vi "3D Drift Control.vi"() -> ()   [LabVIEW 2010]
uses:
  <vilib>/Analysis/NI_AALBase.lvlib
panel:
  out "Boolean":bool
  out "date string":string
  in  "date format (0)":enum16{"short", "long", "abbreviated"}(ring)
  in  "Reset":bool
  in  "# Average":i32=1 min=1 max=20 step=1
  in  "Position (um)":dbl=5.0 min=0.0 max=12.0 format="%0.2f"
  in  "Center Piezo":bool
  in  "reset":bool
  out "?":bool
  in  "autofocus":bool
  out "afTemplateImg":dbl[][](array[numeric])
  in  "Select Lockin \n(autofocus)":bool
  out "Image":u8[][](graph)
  out "ztemplateImg":dbl[][](array[numeric])
  in  "z-template":dbl=0.8
  out "z-sensitivity":dbl
  in  "P (z)":dbl=0.1
  in  "I (z)":dbl=0.0005
  out "z-setpoint":dbl
  in  "z-window (um)":dbl=0.5
  in  "z-stepsiz (um)":dbl=0.1
  out "Step":i32
  in  "Save Data":bool
  out "Total Steps":dbl
  in  "stop":bool
  in  "Exposure time 2":dbl(slide)=16.823708333333332 min=0.06254166666666666 max=66.66941666666666 step=0.06254166666666666 scale=0.06254166666666666..103.94425 scale format="%#.3g"
  in  "Pixel clock":i32(slide)=24 min=5 max=40 scale=5.0..40.0
  in  "Frame rate":dbl(slide)=50.0 min=0.47316940221670395 max=14.999381275522385 step=6.254166666666666e-05 scale=0.47316940221670395..50.0 scale format="%^#_3g"
  in  "?":bool
  in  "pixels2um":dbl=9.8472
  in  "fix z":bool
  in  "fix y":bool
  in  "fix x":bool
  in  "I (xy)":dbl=0.0005
  in  "P (xy)":dbl=0.1
  out "# of frames":i32
  out "?":cluster{"Y":dbl[], "Y":dbl[]}[](graph)
  in  "Monitor Drift":bool
  out "status":dbl
  out "lockinImg":dbl[][](array[numeric])
  out "centery":dbl
  out "centerx":dbl
  out "?":bool
  in  "Select Lockin\n(Drift Bead)":bool
  in  "templateSiz":dbl=50.0
  in  "add Factor":dbl=20.0
  in  "scale":dbl=9.0
  in  "Filename":string="Drift"
  in  "Index #":i32=1
  out "X Position":dbl
  out "Y Position":dbl
  out "Z Position":dbl
  # "drift"
  # "autofocus"
  # "O"
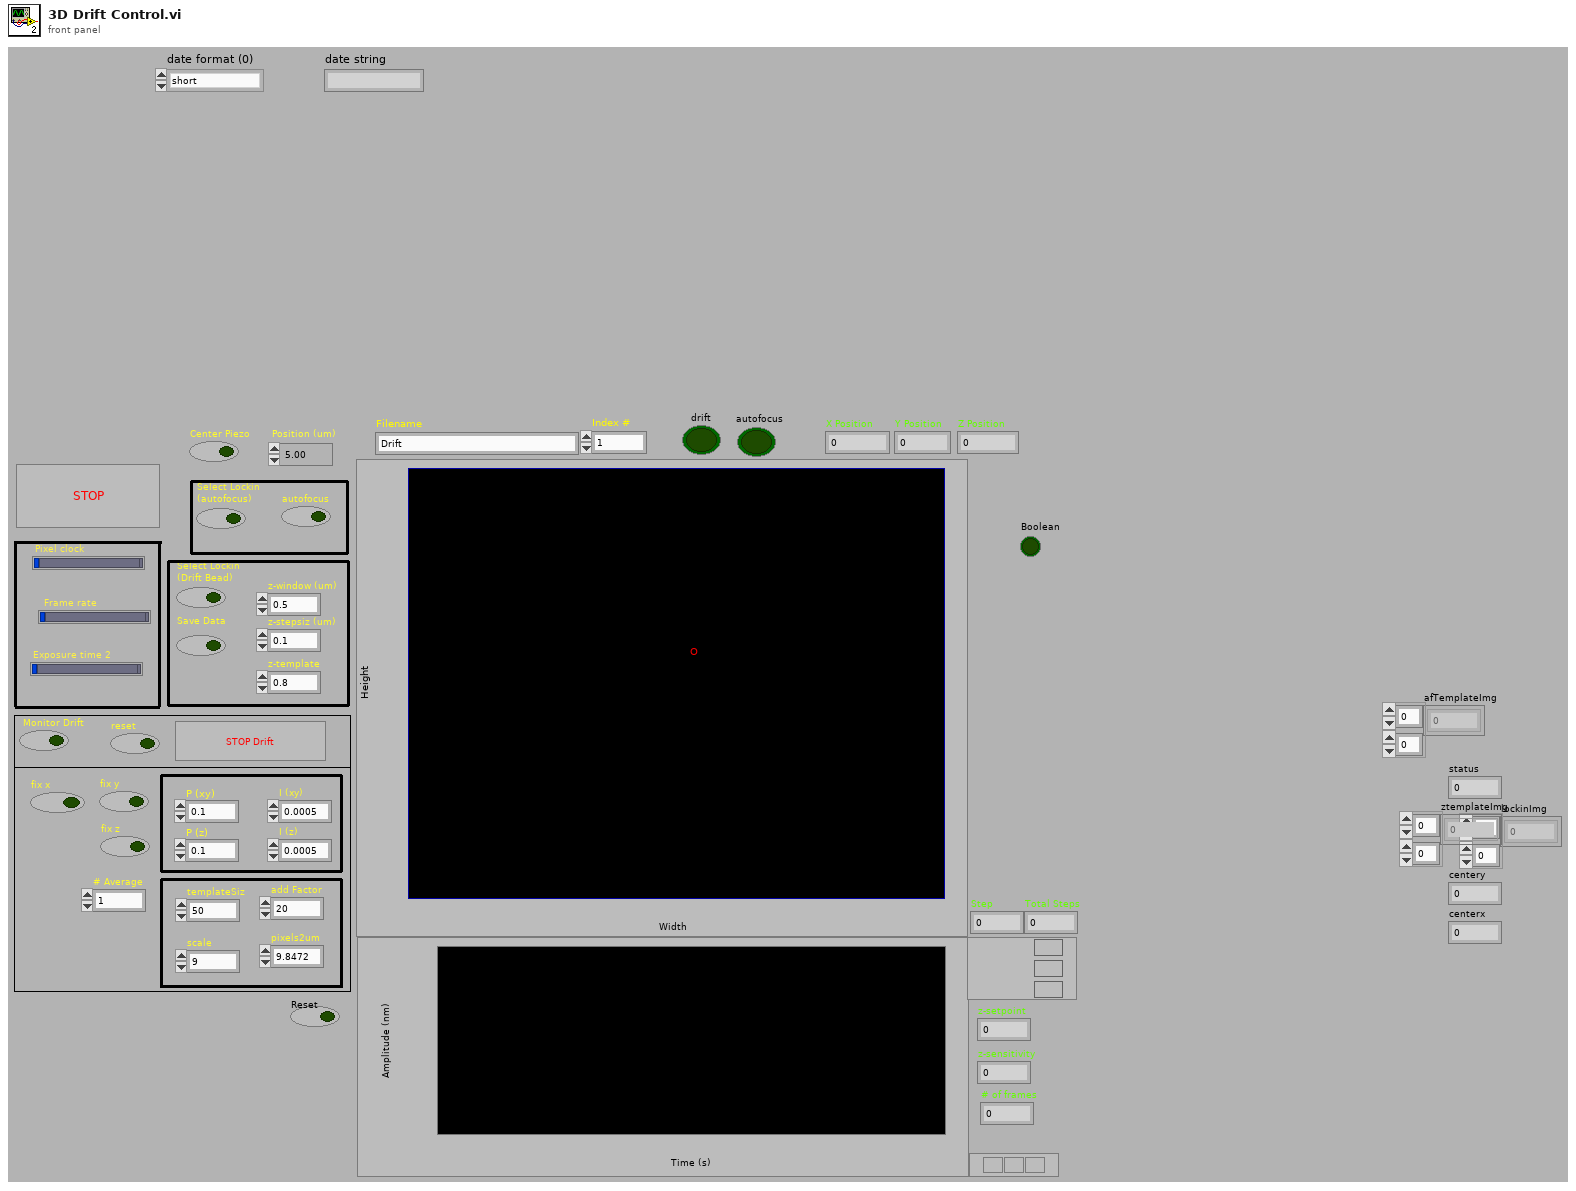
[diagram p1: front panel]
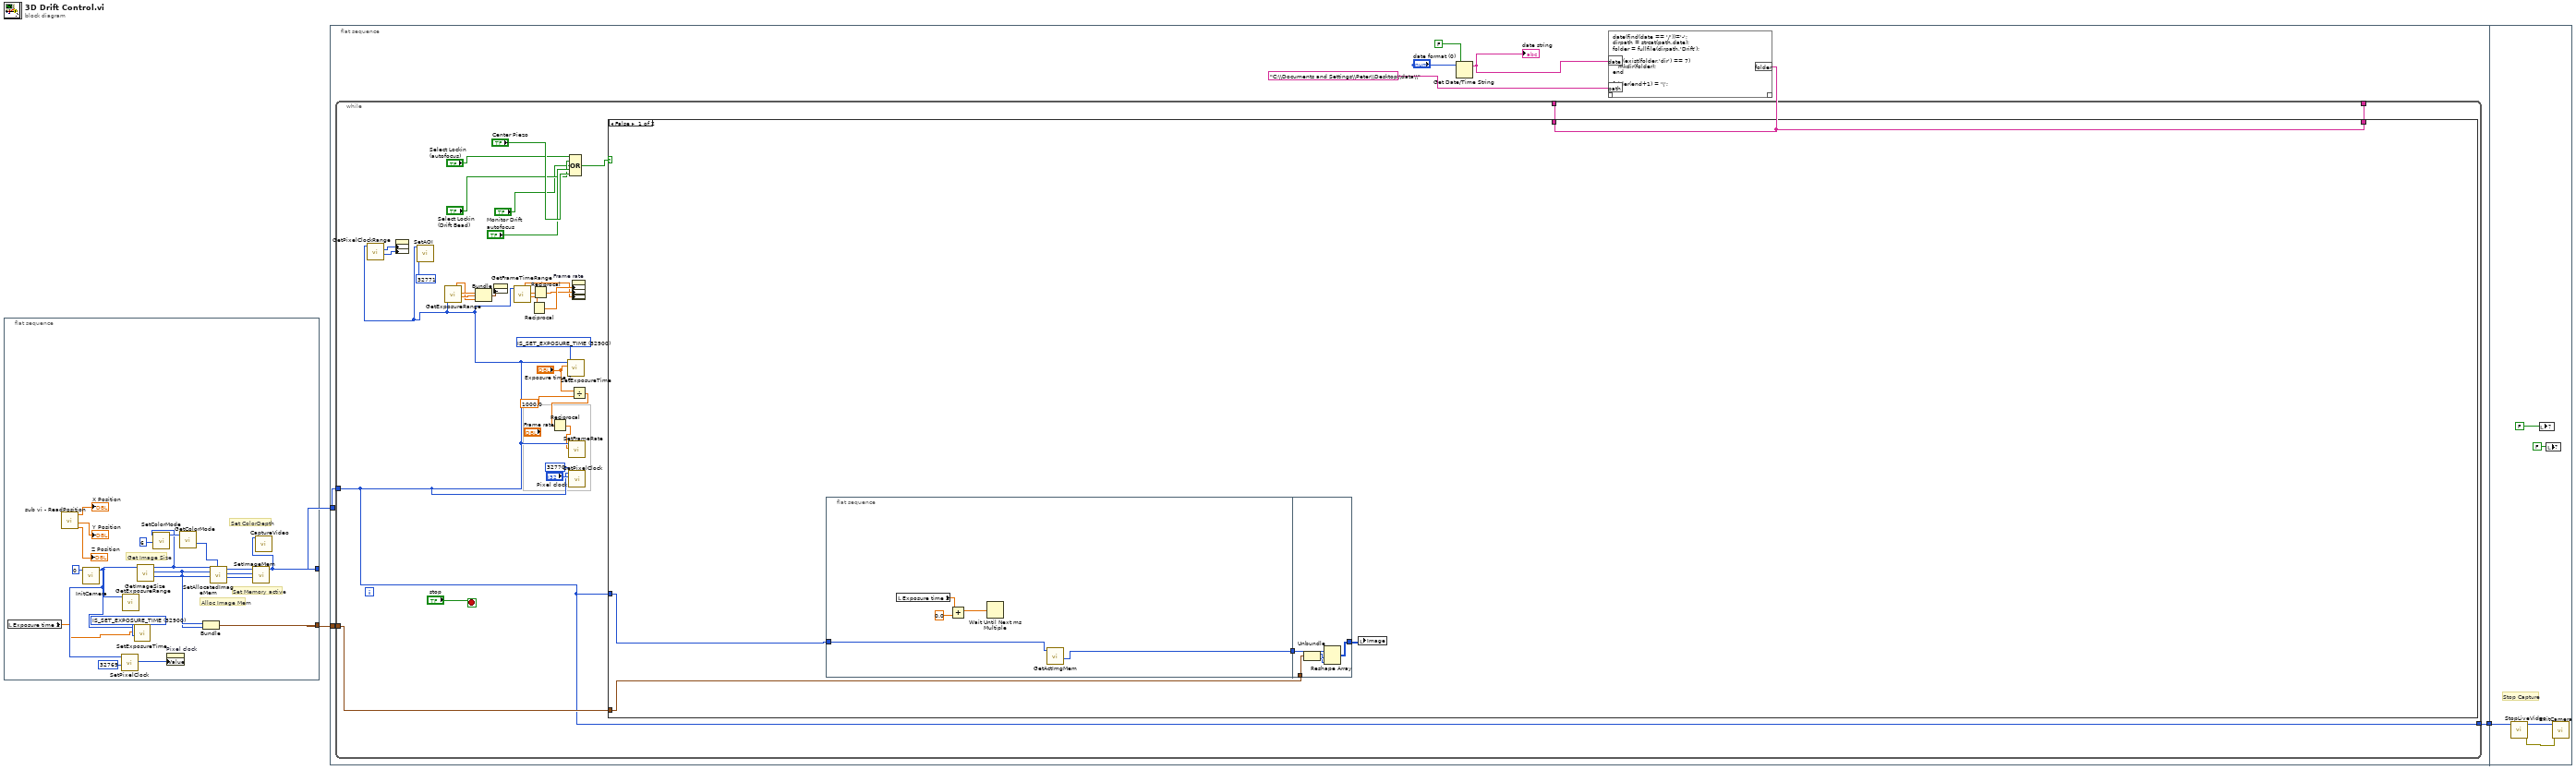
[diagram p0: block diagram]
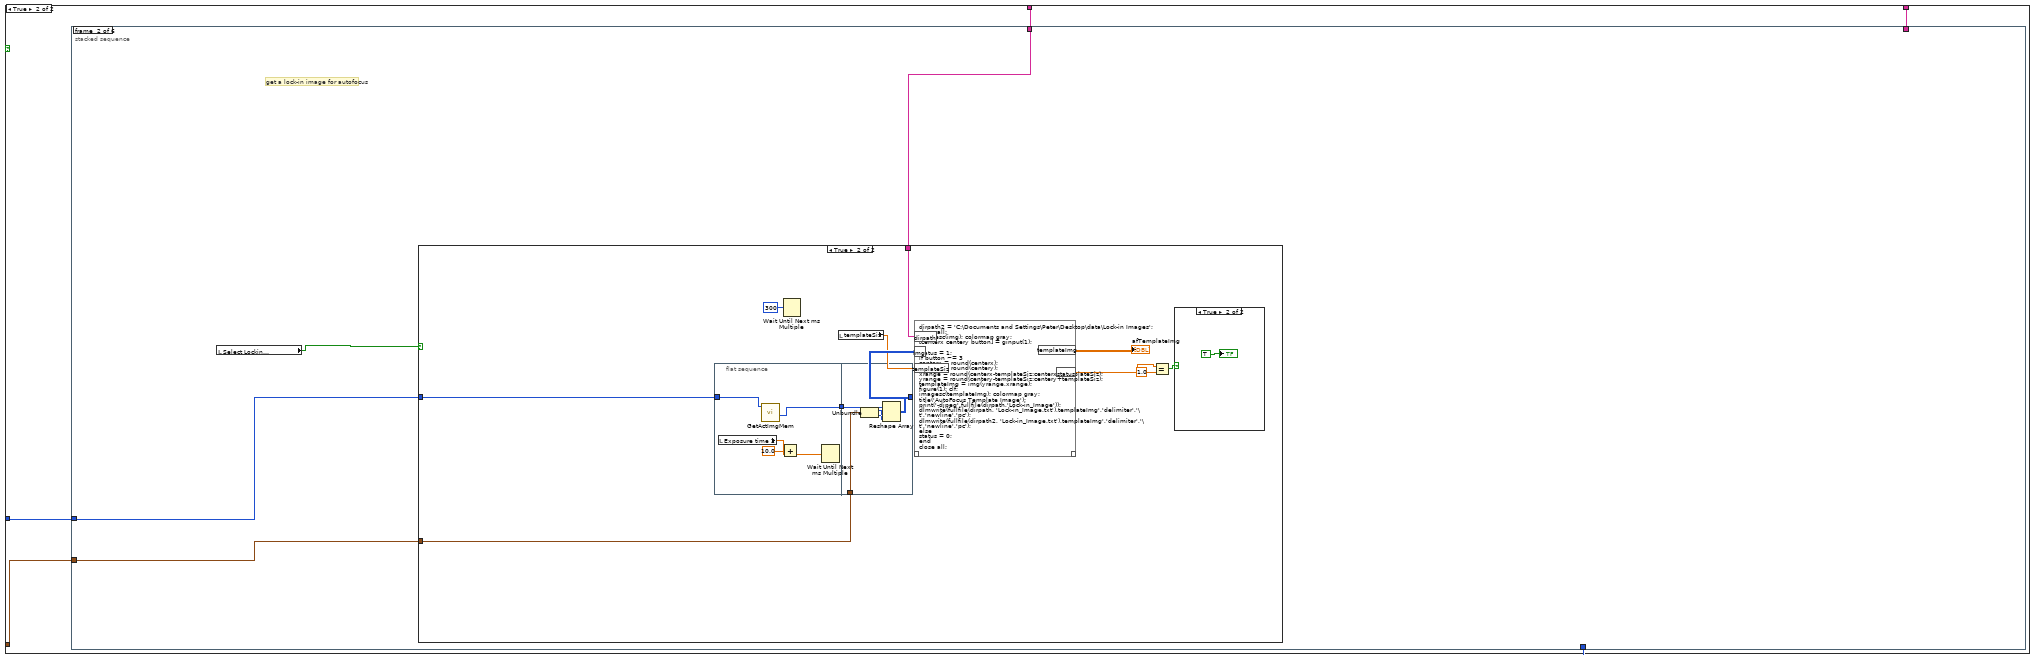
[diagram p2: hidden frame]
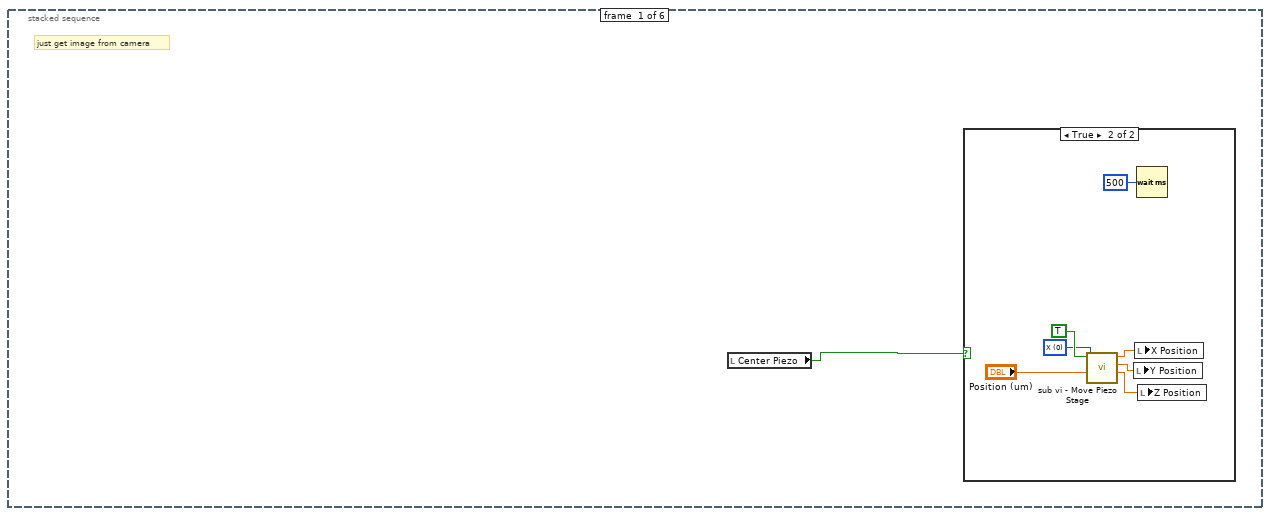
[diagram p3: hidden frame]
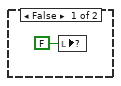
[diagram p6: hidden frame]
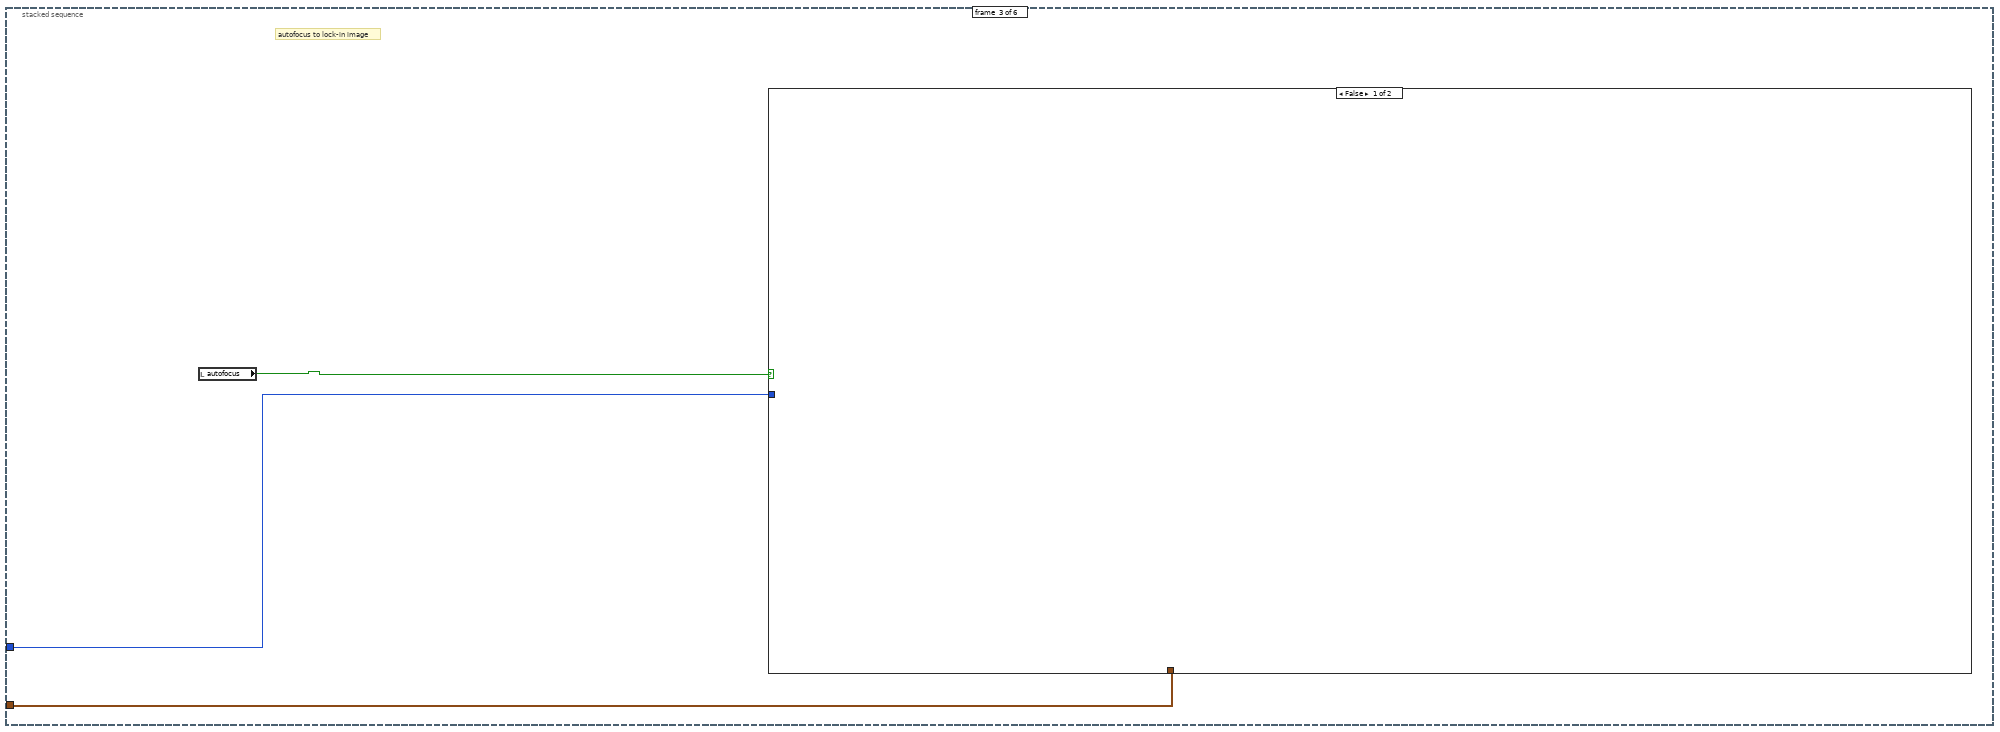
[diagram p7: hidden frame]
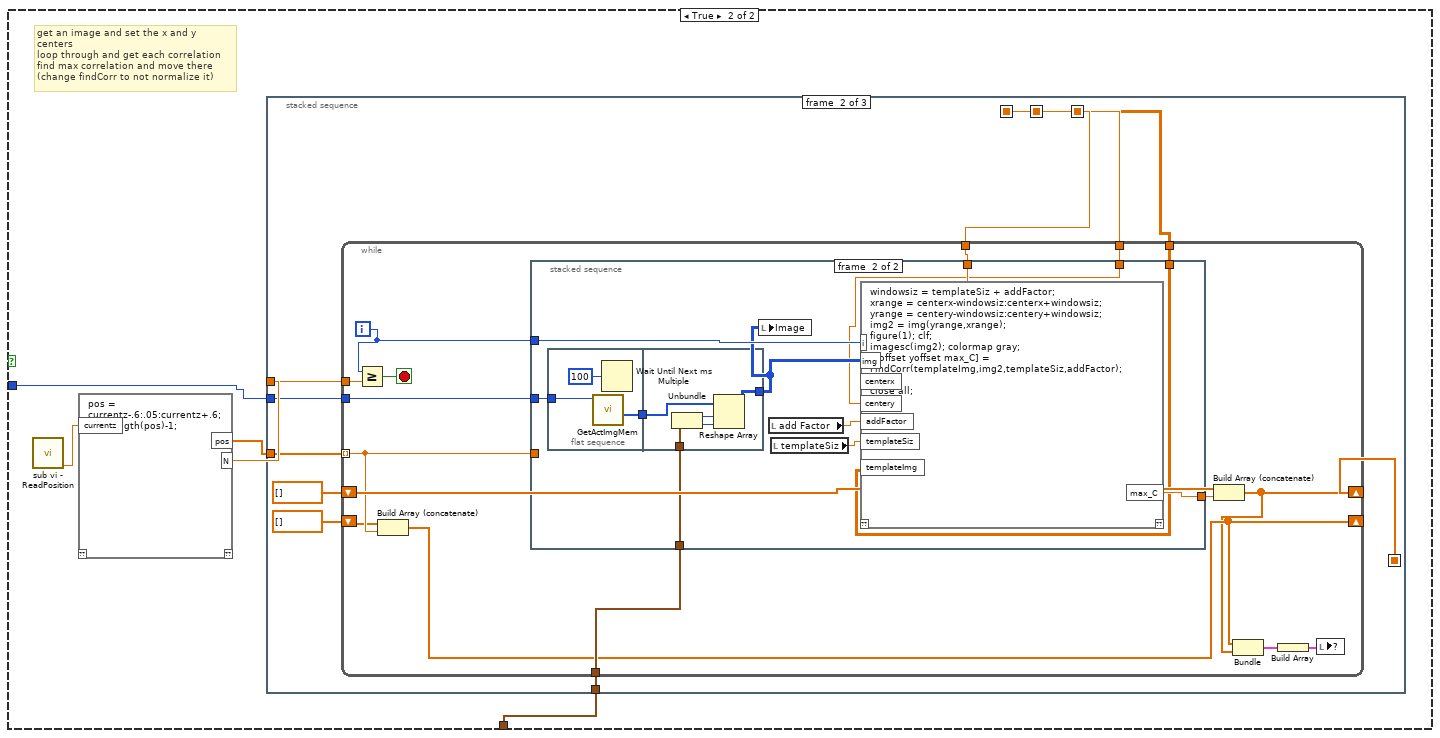
[diagram p8: hidden frame]
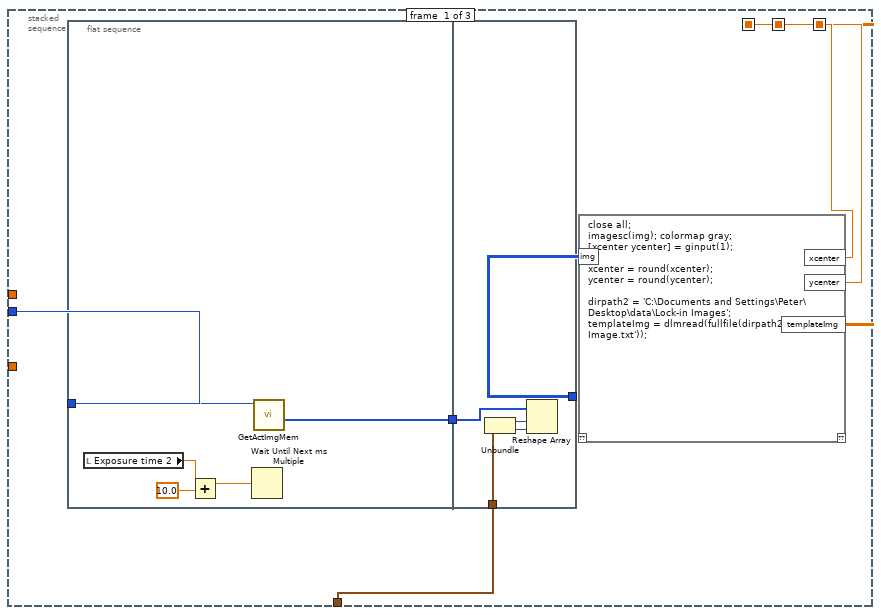
[diagram p9: hidden frame]
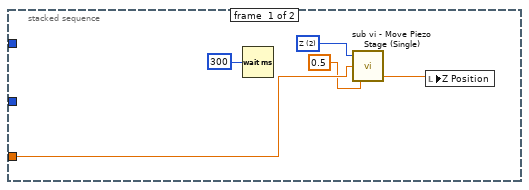
[diagram p10: hidden frame]
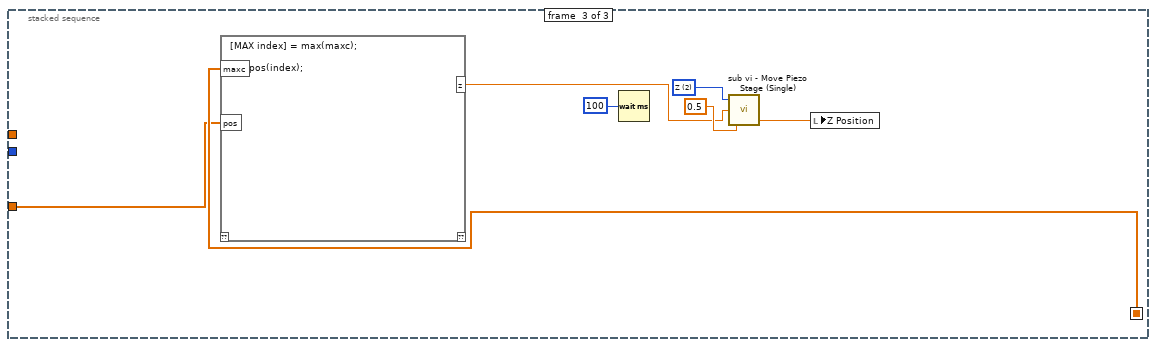
[diagram p11: hidden frame]
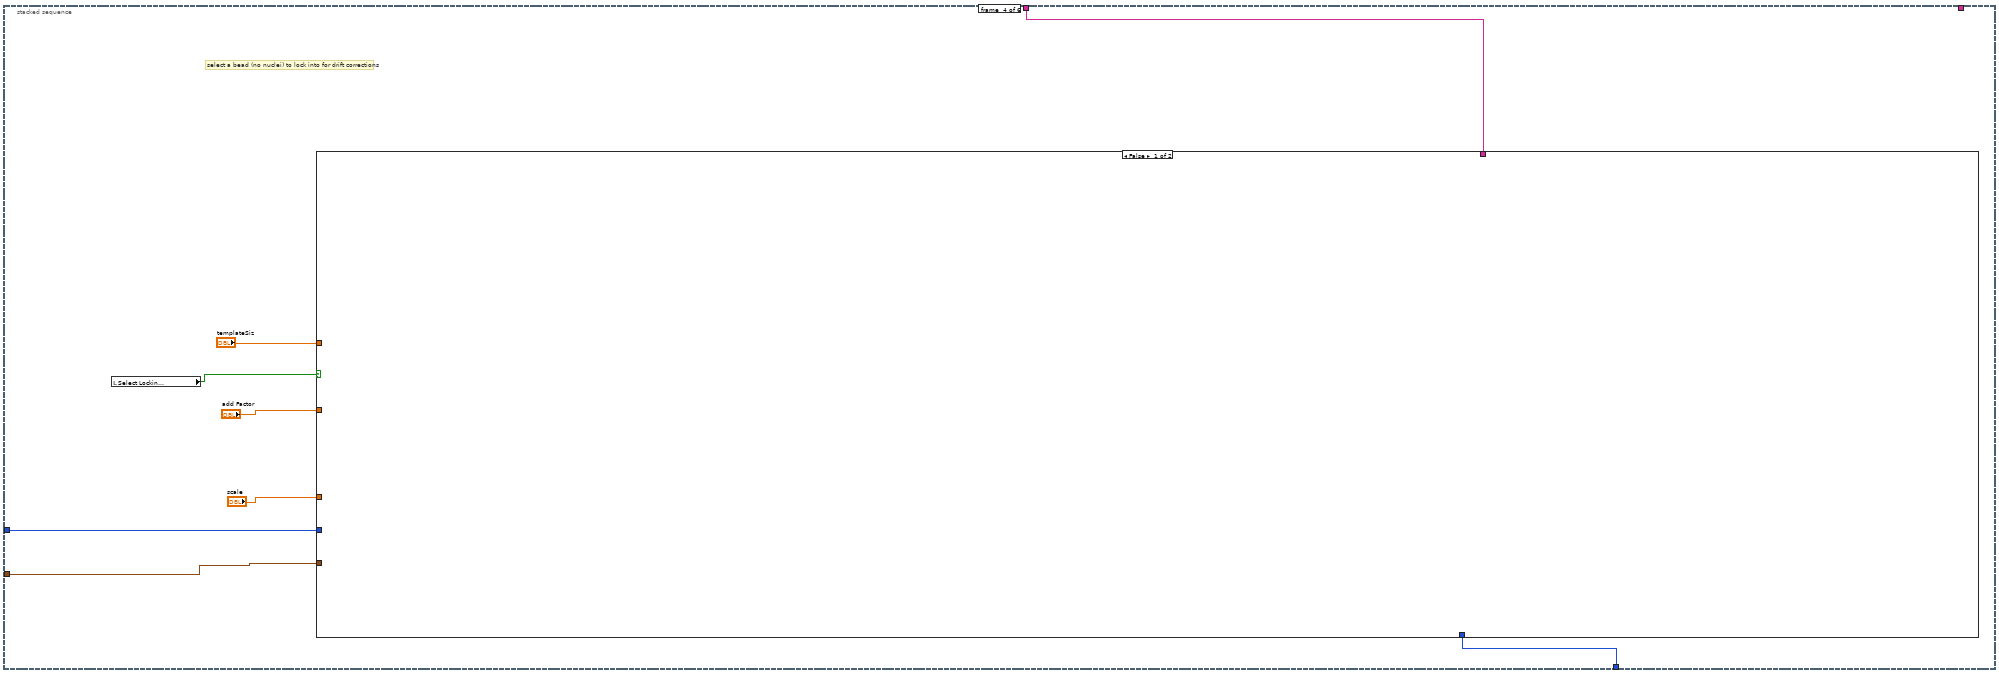
[diagram p12: hidden frame]
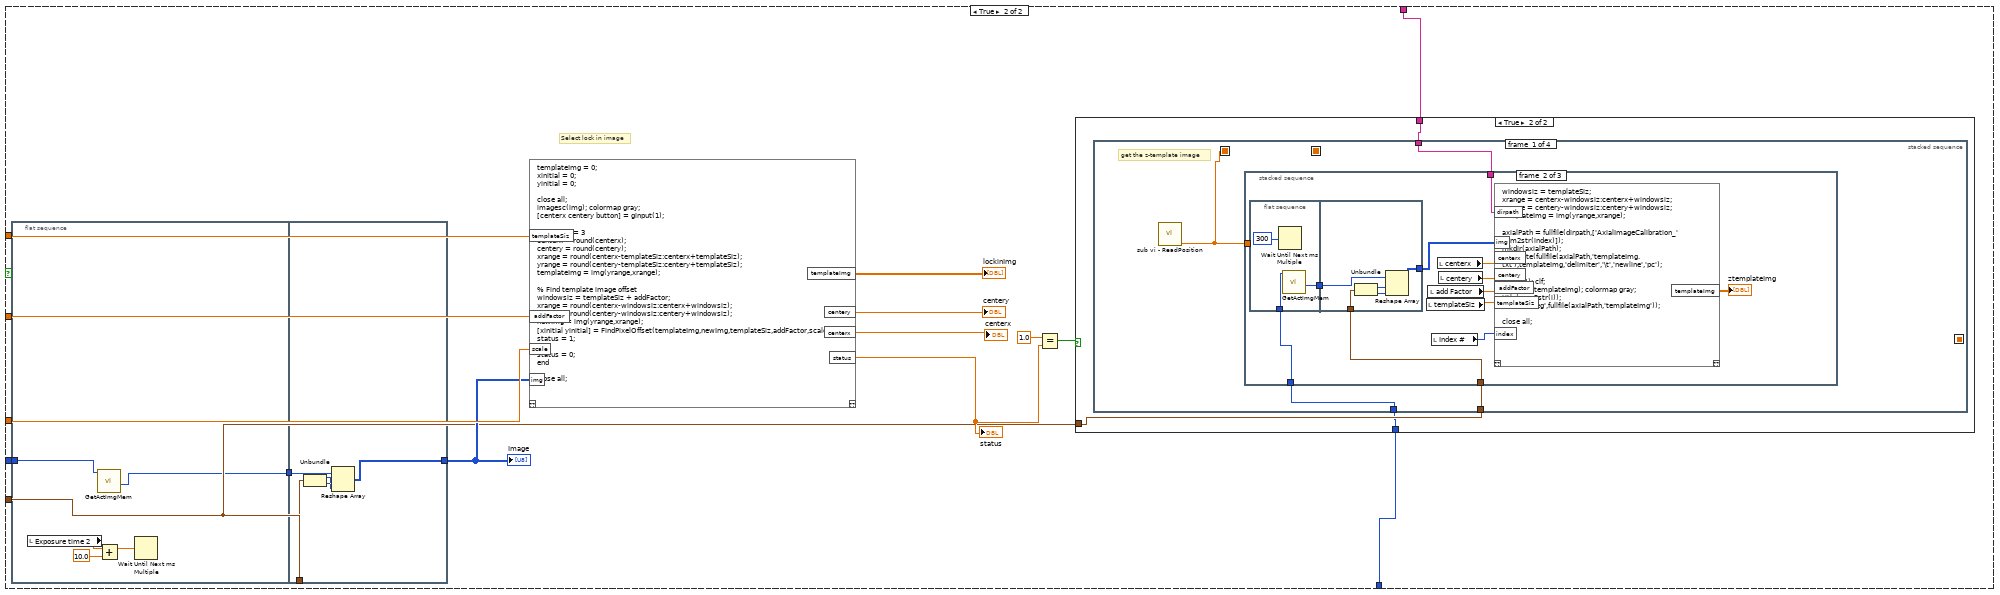
[diagram p13: hidden frame]
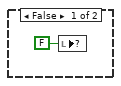
[diagram p14: hidden frame]
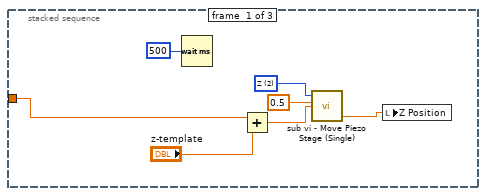
[diagram p15: hidden frame]
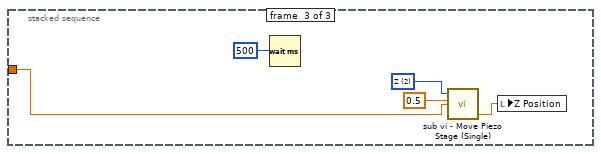
[diagram p16: hidden frame]
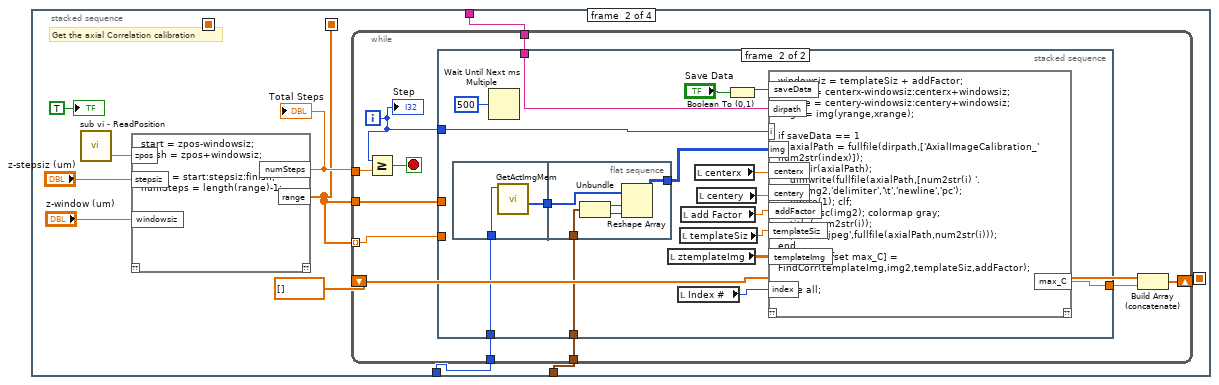
[diagram p17: hidden frame]
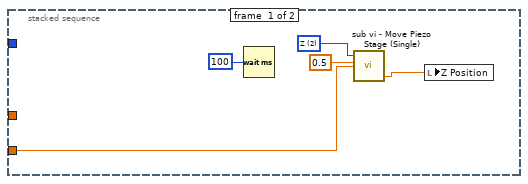
[diagram p18: hidden frame]
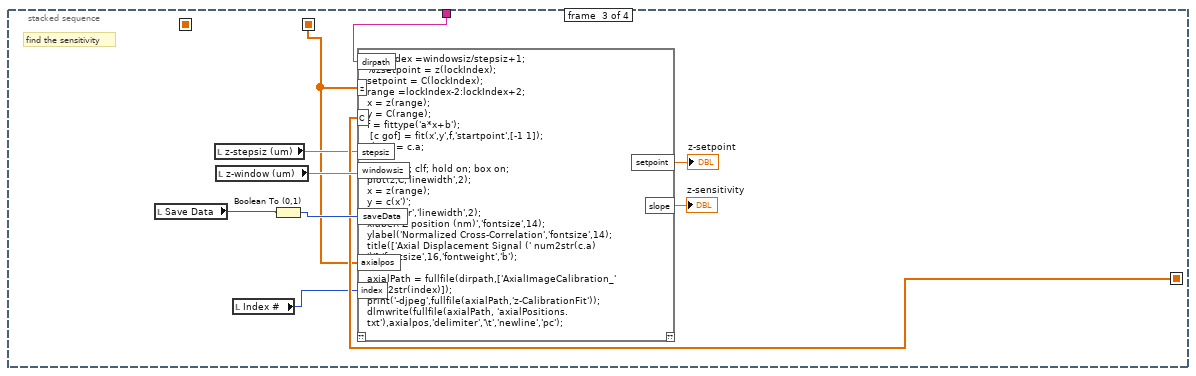
[diagram p19: hidden frame]
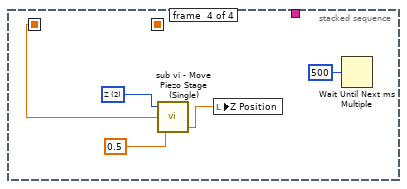
[diagram p20: hidden frame]
diagram:
  n1 = flat-sequence {
    tunnel: [w6] -> w2
    tunnel: [w9] -> w1
    frame #0 {
      w11 = u16 32900 items=["IS_SET_EXPOSURE_TIME"=32900, "IS_GET_EXPOSURE_TIME"=32768, "IS_GET_DEFAULT_EXPOSURE"=32769] ("Mode")
      # "Set Memory active"
      # "Alloc Image Mem"
      # "Set ColorDepth"
      # "Get Image Size"
      n2 = local read "Exposure time 2"() -> (w7:dbl)
      n3 = call "sub vi - ReadPosition.vi"() -> ("Z Position"=→"Z Position":dbl, "Y Position"=→"Y Position":dbl, "X Position"=→"X Position":dbl)  [unwired: 6 in, 3 out]
      n4 = call "InitCamera.vi"("Camera ID"=u32 0) -> ("Camera Handle Out"=w10:u32)  [unwired: 10 out]
      n5 = call "SetPixelClock.vi"("Mode"=32769, "Camera Handle In"=w10) -> ("Value"=w8:i32)  [unwired: 2 in, 7 out]
      n6 = call "GetExposureRange.vi"("Camera Handle In"=w10) -> ()  [unwired: 1 in, 10 out]
      n7 = call "SetExposureTime.vi"("Mode"=w11, "Exposure Time"=w7, "Camera Handle In"=w10) -> ()  [unwired: 2 in, 7 out]
      n8 = call "GetImageSize.vi"("Camera Handle In"=w10) -> ("Height"=w13:i32, "Width"=w12:i32, "Camera Handle Out"=w4:u32)  [unwired: 8 out]
      n9 = call "SetColorMode.vi"("Mode"=6, "Camera Handle In"=w4) -> ("Camera Handle Out"=w16:u32)  [unwired: 1 in, 8 out]
      n10 = property on="Pixel clock" class="Slide (strict)"("Value"=w8) -> ()  [unwired: 2 in, 2 out]
      n11 = call "GetColorMode.vi"("Camera Handle In"=w16) -> ("Bits/Pixel"=w14:i32)  [unwired: 10 out]
      n12 = Bundle("Height"=w13, "Width"=w12) -> (w9:cluster{"Height":i32, "Width":i32})  [unwired: 1 out]
      n13 = call "SetAllocatedImageMem.vi"("BitsPixel"=w14, "Height"=w13, "Width"=w12, "Camera Handle In"=w4) -> ("Image Memory Out"=w18:u8[], "Memory ID Out"=w19:i32, "Camera Handle Out"=w20:u32)  [unwired: 1 in, 4 out]
      n14 = call "SetImageMem.vi"("Image Memory In"=w18, "Memory ID In"=w19, "Camera Handle In"=w20) -> ("Camera Handle Out"=w6:u32)  [unwired: 1 in, 7 out]
      n15 = call "CaptureVideo.vi"("Camera Handle In"=w6) -> ()  [unwired: 2 in, 9 out]
    }
  }
  n16 = flat-sequence {
    tunnel: w2 -> [w31]
    tunnel: w1 -> [w30]
    tunnel: [w29] -> w3
    tunnel: w3 -> [w558]
    frame #0 {
      n17 = Get Date/Time String(date format (0)="date format (0)", want seconds? (F)=FALSE) -> (date string=w26:string)  [unwired: 2 out]
      "date string" <- w26
      n18 = script code="date(find(date == '/'))='-';\ndirpath = strcat(path,date);\nfolder = fullfile(dirpath,'Drift');\n\nif ~(exist(folder,'dir') == 7)\n   mkdir(folder);\nend\n\nfolder(end+1) = '\\';"("date"=w26, "path"="C:\\Documents and Settings\\Peter\\Desktop\\data\\" ("String")) -> ("folder"=w24:string)  [unwired: 2 out]
      n19 = while {
        tunnel: w31 -> [w42]
        tunnel: w30 -> [w57]
        tunnel: [w42] -> w29
        tunnel: w24 -> [w56]
        tunnel: w24 -> [w55]
        stop <- "stop" stop-if-true
        w59 = u16 32900 items=["IS_SET_EXPOSURE_TIME"=32900, "IS_GET_EXPOSURE_TIME"=32768, "IS_GET_DEFAULT_EXPOSURE"=32769] ("Mode")
        n20 = call "GetPixelClockRange.vi"("Camera Handle In"=w42) -> ("Max"=w54:i32, "Min"=w53:i32)  [unwired: 1 in, 8 out]
        n21 = property on="Pixel clock" class="Schieberegler (strikt)"("Minimum"=w53, "Maximum"=w54) -> ()  [unwired: 2 in, 2 out]
        n22 = call "SetAOI.vi"("Camera Handle In"=w42, "Mode"=32771) -> ()  [unwired: 5 in, 9 out]
        n23 = call "GetExposureRange.vi"("Camera Handle In"=w42) -> ("max"=w49:dbl, "min"=w50:dbl, "intervall"=w48:dbl)  [unwired: 1 in, 7 out]
        n24 = Bundle("min"=w50, "max"=w49, "intervall"=w48) -> (w51:cluster{"min":dbl, "max":dbl, "intervall":dbl})  [unwired: 1 out]
        n25 = property on="Exposure time 2" class="Schieberegler (strikt)"("Data Range"=w51) -> ()  [unwired: 2 in, 2 out]
        n26 = call "GetFrameTimeRange.vi"("Camera Handle In"=w42) -> ("max"=w47:dbl, "min"=w46:dbl, "interval"=w43:dbl)  [unwired: 1 in, 7 out]
        n27 = Reciprocal(x=w47) -> (1/x=w45:dbl)
        n28 = Reciprocal(x=w46) -> (1/x=w44:dbl)
        n29 = call "SetExposureTime.vi"("Mode"=w59, "Exposure Time"="Exposure time 2", "Camera Handle In"=w42) -> ()  [unwired: 1 in, 8 out]
        n30 = call "SetPixelClock.vi"("Mode"=32770, "Pixel Clock"="Pixel clock", "Camera Handle In"=w42) -> ()  [unwired: 1 in, 8 out]
        n31 = Compound Arithmetic op=OR("Select Lockin \n(autofocus)", "Select Lockin\n(Drift Bead)", "Monitor Drift", "autofocus", "Center Piezo") -> (w37:bool)
        n32 = Divide(x="Exposure time 2", y=1000.0) -> (x/y=w38:dbl)
        n33 = Reciprocal(x=w38) -> (1/x=w41:dbl)
        n34 = call "SetFrameRate.vi"("FPS"=w41, "Camera Handle In"=w42) -> ()  [unwired: 1 in, 9 out]
        n35 = property on="Frame rate" class="Schieberegler (strikt)"("Minimum"=w45, "Maximum"=w44, "Increment"=w43) -> ()  [unwired: 2 in, 2 out]
        n36 = case shown="False" w37 {
          tunnel: w57 -> [w62 w79]
          tunnel: w56 -> [_ w78]
          tunnel: w55 -> [_ w77]
          tunnel: w42 -> [w63 w76]
          frame False {
            n37 = flat-sequence {
              tunnel: [w70] -> w65
              tunnel: w63 -> [w66]
              tunnel: w65 -> [w75]
              tunnel: w62 -> [w74]
              tunnel: [w71] -> w64
              frame #0 {
                n38 = local read "Exposure time 2"() -> (w69:dbl)
                n39 = Add(x=w69, y=0.0) -> (x+y=w68:dbl)
                n40 = Wait Until Next ms Multiple(millisecond multiple=w68) -> ()  [unwired: 1 out]
                n41 = call "GetActImgMem.vi"("Camera Handle In"=w66) -> ("Image Memory Out"=w70:u8[])  [unwired: 1 in, 9 out]
              }
              frame #1 {
                n42 = Unbundle(w74) -> ("Height"=w73:i32, "Width"=w72:i32)
                n43 = Reshape Array(w75, w73, w72) -> (w71:u8[][])
              }
            }
            n44 = local write "Image"(w64) -> ()
          }
          frame True {
            n45 = stacked-sequence {
              tunnel: w76 -> [_ w91 w116 w198 w339 _]
              tunnel: w79 -> [_ w90 w117 w199 w340 _]
              tunnel: w78 -> [_ w89 _ w201 _ _]
              tunnel: w76 -> [_ _ _ w200 _ _]
              tunnel: w77 -> [_ _ _ _ w335 _]
              frame #0 {
                # "just get image from camera"
                n46 = local read "Center Piezo"() -> (w80:bool)
                n47 = case shown="True" w80 {
                  frame False {
                  }
                  frame True {
                    w86 = u16 0 items=["X", "Y", "Z"] ("Axis")
                    n48 = call "sub vi - Move Piezo Stage.vi"("Desired Position (um)"="Position (um)", "Axis"=w86, "All Axis"=TRUE) -> ("Z Position"=w83:dbl, "Y Position"=w84:dbl, "X Position"=w85:dbl)  [unwired: 6 in]
                    n49 = local write "Y Position"(w84) -> ()
                    n50 = local write "X Position"(w85) -> ()
                    n51 = Wait (ms)(milliseconds to wait=u32 500) -> ()  [unwired: 1 out]
                    n52 = local write "Z Position"(w83) -> ()
                  }
                }
              }
              frame #1 {
                # "get a lock-in image for autofocus"
                n53 = local read "Select Lockin \n(autofocus)"() -> (w88:bool)
                n54 = case shown="True" w88 {
                  tunnel: w91 -> [_ w101]
                  tunnel: w90 -> [_ w100]
                  tunnel: w89 -> [_ w99]
                  frame False {
                  }
                  frame True {
                    n55 = flat-sequence {
                      tunnel: [w109] -> w102
                      tunnel: w101 -> [w108]
                      tunnel: w102 -> [w114]
                      tunnel: w100 -> [w113]
                      tunnel: [w110] -> w98
                      frame #0 {
                        n56 = local read "Exposure time 2"() -> (w107:dbl)
                        n57 = call "GetActImgMem.vi"("Camera Handle In"=w108) -> ("Image Memory Out"=w109:u8[])  [unwired: 1 in, 9 out]
                        n58 = Add(x=10.0, y=w107) -> (x+y=w106:dbl)
                        n59 = Wait Until Next ms Multiple(millisecond multiple=w106) -> ()  [unwired: 1 out]
                      }
                      frame #1 {
                        n60 = Unbundle(w113) -> ("Height"=w112:i32, "Width"=w111:i32)
                        n61 = Reshape Array(w114, w112, w111) -> (w110:u8[][])
                      }
                    }
                    n62 = Wait Until Next ms Multiple(millisecond multiple=u32 300) -> ()  [unwired: 1 out]
                    n63 = local read "templateSiz"() -> (w96:dbl)
                    n64 = script code="dirpath2 = 'C:\\Documents and Settings\\Peter\\Desktop\\data\\Lock-in Images';\nclose all;\nimagesc(img); colormap gray;\n[centerx centery button] = ginput(1);\n\nstatus = 1;\nif button ~= 3\ncenterx = round(centerx);\ncentery = round(centery);\nxrange = round(centerx-templateSiz:centerx+templateSiz);\nyrange = round(centery-templateSiz:centery+templateSiz);\ntemplateImg = img(yrange,xrange);\nfigure(1); clf;\nimagesc(templateImg); colormap gray;\ntitle('AutoFocus Template Image');\nprint('-djpeg',fullfile(dirpath,'Lock-in_Image'));\ndlmwrite(fullfile(dirpath, 'Lock-in_Image.txt'),templateImg','delimiter','\\t','newline','pc');\ndlmwrite(fullfile(dirpath2, 'Lock-in_Image.txt'),templateImg','delimiter','\\t','newline','pc');\nelse\nstatus = 0;\nend\nclose all;"("dirpath"=w99, "img"=w98, "templateSiz"=w96) -> ("templateImg"=→"afTemplateImg":dbl[][], "status"=w94:dbl)  [unwired: 1 in, 1 out]
                    n65 = Equal?(x=w94, y=1.0) -> (x = y?=w93:bool)
                    n66 = case shown="True" w93 {
                      frame False {
                        n67 = local write item#43(FALSE) -> ()
                      }
                      frame True {
                        "?" <- TRUE
                      }
                    }
                  }
                }
              }
              frame #2 {
                # "autofocus to lock-in image"
                n68 = local read "autofocus"() -> (w115:bool)
                n69 = case shown="False" w115 {
                  tunnel: w117 -> [_ w122]
                  tunnel: w116 -> [_ w121]
                  frame False {
                  }
                  frame True {
                    # "get an image and set the x and y centers\nloop through and get each correlation\nfind max correlation and move there\n(change findCorr to not normalize it)"
                    n70 = call "sub vi - ReadPosition.vi"() -> ("Z Position"=w120:dbl)  [unwired: 6 in, 5 out]
                    n71 = script code="pos = currentz-.6:.05:currentz+.6;\nN = length(pos)-1;"("currentz"=w120) -> ("pos"=w119:dbl[], "N"=w118:dbl)  [unwired: 1 in, 1 out]
                    n72 = stacked-sequence {
                      seq-local: [w125 _ _] -> [_ w145 _]
                      seq-local: [w124 _ _] -> [_ w144 _]
                      seq-local: [_ w143 _] -> [_ _ w196]
                      seq-local: [w123 _ _] -> [_ w140 _]
                      tunnel: w122 -> [w128 w149 _]
                      tunnel: w121 -> [w127 w148 _]
                      tunnel: w119 -> [_ w147 w195]
                      tunnel: w118 -> [_ w146 _]
                      frame #0 {
                        n73 = flat-sequence {
                          tunnel: [w134] -> w129
                          tunnel: w127 -> [w133]
                          tunnel: w129 -> [w139]
                          tunnel: [w138] -> w126
                          tunnel: w128 -> [w137]
                          frame #0 {
                            n74 = local read "Exposure time 2"() -> (w132:dbl)
                            n75 = Add(x=w132, y=10.0) -> (x+y=w131:dbl)
                            n76 = Wait Until Next ms Multiple(millisecond multiple=w131) -> ()  [unwired: 1 out]
                            n77 = call "GetActImgMem.vi"("Camera Handle In"=w133) -> ("Image Memory Out"=w134:u8[])  [unwired: 1 in, 9 out]
                          }
                          frame #1 {
                            n78 = Unbundle(w137) -> ("Height"=w136:i32, "Width"=w135:i32)
                            n79 = Reshape Array(w139, w136, w135) -> (w138:u8[][])
                          }
                        }
                        n80 = script code="close all;\nimagesc(img); colormap gray;\n[xcenter ycenter] = ginput(1);\n\nxcenter = round(xcenter);\nycenter = round(ycenter);\n\ndirpath2 = 'C:\\Documents and Settings\\Peter\\Desktop\\data\\Lock-in Images';\ntemplateImg = dlmread(fullfile(dirpath2, 'Lock-in_Image.txt'));"("img"=w126) -> ("xcenter"=w125:dbl, "ycenter"=w124:dbl, "templateImg"=w123:dbl[][])  [unwired: 1 in, 1 out]
                      }
                      frame #1 {
                        n81 = while {
                          shift-right: [w153] -> w143
                          shift-left: dbl[] [] -> [w162]
                          tunnel: w149 -> [w161]
                          tunnel: w148 -> [w160]
                          tunnel: w147 -> [w156] mode=indexing
                          tunnel: w146 -> [w159]
                          tunnel: w145 -> [w158]
                          tunnel: w144 -> [w157]
                          shift-right: [w154] -> _
                          shift-left: dbl[] [] -> [w155]
                          tunnel: w140 -> [w150]
                          i -> [w165]
                          stop <- w164 stop-if-true
                          n82 = Greater Or Equal?(x=w165, y=w159) -> (x >= y?=w164:bool)
                          n83 = Build Array (concatenate)(w155, w156) -> (w154:dbl[])
                          n84 = stacked-sequence {
                            tunnel: w165 -> [_ w180]
                            tunnel: [_ w179] -> w163
                            tunnel: w161 -> [_ w177]
                            tunnel: w160 -> [_ w176]
                            tunnel: w156 -> [w168 _]
                            tunnel: w158 -> [_ w173]
                            tunnel: w157 -> [_ w172]
                            tunnel: w150 -> [_ w171]
                            frame #0 {
                              w169 = u16 2 items=["X", "Y", "Z"] ("Axis")
                              n85 = Wait (ms)(milliseconds to wait=u32 300) -> ()  [unwired: 1 out]
                              n86 = call "sub vi - Move Piezo Stage (Single).vi"("frequency"=0.5, "Desired Position (um)"=w168, "Axis"=w169) -> ("Z Position"=w166:dbl)  [unwired: 2 out]
                              n87 = local write "Z Position"(w166) -> ()
                            }
                            frame #1 {
                              n88 = flat-sequence {
                                tunnel: [w184] -> w181
                                tunnel: w176 -> [w183]
                                tunnel: w181 -> [w189]
                                tunnel: [w188] -> w178
                                tunnel: w177 -> [w187]
                                frame #0 {
                                n89 = call "GetActImgMem.vi"("Camera Handle In"=w183) -> ("Image Memory Out"=w184:u8[])  [unwired: 1 in, 9 out]
                                n90 = Wait Until Next ms Multiple(millisecond multiple=u32 100) -> ()  [unwired: 1 out]
                                }
                                frame #1 {
                                n91 = Unbundle(w187) -> ("Height"=w186:i32, "Width"=w185:i32)
                                n92 = Reshape Array(w189, w186, w185) -> (w188:u8[][])
                                }
                              }
                              n93 = local write "Image"(w178) -> ()
                              n94 = local read "add Factor"() -> (w175:dbl)
                              n95 = local read "templateSiz"() -> (w174:dbl)
                              n96 = script code="windowsiz = templateSiz + addFactor;\nxrange = centerx-windowsiz:centerx+windowsiz;\nyrange = centery-windowsiz:centery+windowsiz;\nimg2 = img(yrange,xrange);\nfigure(1); clf; \nimagesc(img2); colormap gray;\n[xoffset yoffset max_C] = FindCorr(templateImg,img2,templateSiz,addFactor);\n            \nclose all;"("img"=w178, "centerx"=w173, "centery"=w172, "i"=w180, "addFactor"=w175, "templateSiz"=w174, "templateImg"=w171) -> ("max_C"=w179:dbl)  [unwired: 1 in, 1 out]
                            }
                          }
                          n97 = Build Array (concatenate)(w162, w163) -> (w153:dbl[])
                          n98 = Bundle(w154, w153) -> (w152:cluster{dbl[], dbl[]})  [unwired: 1 in]
                          n99 = Build Array(w152) -> (w151:cluster{dbl[], dbl[]}[])
                          n100 = local write item#15(w151) -> ()
                        }
                      }
                      frame #2 {
                        w193 = u16 2 items=["X", "Y", "Z"] ("Axis")
                        n101 = script code="[MAX index] = max(maxc);\n\nz = pos(index);"("maxc"=w196, "pos"=w195) -> ("z"=w191:dbl)  [unwired: 1 in, 1 out]
                        n102 = Wait (ms)(milliseconds to wait=u32 100) -> ()  [unwired: 1 out]
                        n103 = call "sub vi - Move Piezo Stage (Single).vi"("frequency"=0.5, "Desired Position (um)"=w191, "Axis"=w193) -> ("Z Position"=w190:dbl)  [unwired: 2 out]
                        n104 = local write "Z Position"(w190) -> ()
                      }
                    }
                  }
                }
              }
              frame #3 {
                # "select a bead (no nuclei) to lock into for drift corrections"
                n105 = local read "Select Lockin\n(Drift Bead)"() -> (w197:bool)
                n106 = case shown="False" w197 {
                  tunnel: "scale" -> [_ w219]
                  tunnel: "add Factor" -> [_ w218]
                  tunnel: "templateSiz" -> [_ w217]
                  tunnel: w201 -> [_ w210]
                  tunnel: w199 -> [_ w206]
                  tunnel: w200 -> [_ w209]
                  tunnel: w198 -> [_ w205]
                  frame False {
                  }
                  frame True {
                    # "Select lock in image"
                    n107 = flat-sequence {
                      tunnel: [w224] -> w208
                      tunnel: w205 -> [w223]
                      tunnel: w208 -> [w229]
                      tunnel: w206 -> [w228]
                      tunnel: [w225] -> w207
                      frame #0 {
                        n108 = local read "Exposure time 2"() -> (w222:dbl)
                        n109 = call "GetActImgMem.vi"("Camera Handle In"=w223) -> ("Image Memory Out"=w224:u8[])  [unwired: 1 in, 9 out]
                        n110 = Add(x=w222, y=10.0) -> (x+y=w221:dbl)
                        n111 = Wait Until Next ms Multiple(millisecond multiple=w221) -> ()  [unwired: 1 out]
                      }
                      frame #1 {
                        n112 = Unbundle(w228) -> ("Height"=w227:i32, "Width"=w226:i32)
                        n113 = Reshape Array(w229, w227, w226) -> (w225:u8[][])
                      }
                    }
                    n114 = script code="templateImg = 0;\nxinitial = 0;\nyinitial = 0;\n\nclose all;\nimagesc(img); colormap gray;\n[centerx centery button] = ginput(1);\n\nif button ~= 3\ncenterx = round(centerx);\ncentery = round(centery);\nxrange = round(centerx-templateSiz:centerx+templateSiz);\nyrange = round(centery-templateSiz:centery+templateSiz);\ntemplateImg = img(yrange,xrange);\n\n% Find template image offset\nwindowsiz = templateSiz + addFactor;\nxrange = round(centerx-windowsiz:centerx+windowsiz);\nyrange = round(centery-windowsiz:centery+windowsiz);\nnewImg = img(yrange,xrange);\n[xinitial yinitial] = FindPixelOffset(templateImg,newImg,templateSiz,addFactor,scale);\nstatus = 1;\nelse\nstatus = 0;\nend\n\nclose all;"("img"=w207, "templateSiz"=w217, "addFactor"=w218, "scale"=w219) -> ("centerx"=→"centerx":dbl, "centery"=→"centery":dbl, "templateImg"=→"lockinImg":dbl[][], "status"=w211:dbl)  [unwired: 1 in, 1 out]
                    "status" <- w211
                    n115 = Equal?(x=1.0, y=w211) -> (x = y?=w213:bool)
                    n116 = case shown="True" w213 {
                      tunnel: w210 -> [_ w233]
                      tunnel: w206 -> [_ w232]
                      tunnel: w209 -> [_ w231]
                      frame False {
                        n117 = local write item#9(FALSE) -> ()
                      }
                      frame True {
                        n118 = stacked-sequence {
                          seq-local: [_ w270 _ _] -> [_ _ w322 _]
                          seq-local: [_ w269 _ _] -> [_ _ w320 _]
                          seq-local: [w234 _ _ _] -> [_ _ _ w331]
                          tunnel: w233 -> [w237 w274 w327 _]
                          tunnel: w232 -> [w235 w273 _ _]
                          tunnel: w231 -> [w236 w272 _ _]
                          frame #0 {
                            # "get the z-template image"
                            n119 = call "sub vi - ReadPosition.vi"() -> ("Z Position"=w234:dbl)  [unwired: 6 in, 5 out]
                            n120 = stacked-sequence {
                              tunnel: w237 -> [_ w253 _]
                              tunnel: w236 -> [_ w248 _]
                              tunnel: w235 -> [_ w247 _]
                              tunnel: w234 -> [w240 _ w266]
                              frame #0 {
                                w243 = u16 2 items=["X", "Y", "Z"] ("Axis")
                                n121 = Wait (ms)(milliseconds to wait=u32 500) -> ()  [unwired: 1 out]
                                n122 = Add(x=w240, y="z-template") -> (x+y=w238:dbl)
                                n123 = call "sub vi - Move Piezo Stage (Single).vi"("frequency"=0.5, "Desired Position (um)"=w238, "Axis"=w243) -> ("Z Position"=w241:dbl)  [unwired: 2 out]
                                n124 = local write "Z Position"(w241) -> ()
                              }
                              frame #1 {
                                n125 = flat-sequence {
                                tunnel: [w258] -> w255
                                tunnel: w248 -> [w257]
                                tunnel: w255 -> [w263]
                                tunnel: [w262] -> w254
                                tunnel: w247 -> [w261]
                                frame #0 {
                                n126 = Wait Until Next ms Multiple(millisecond multiple=u32 300) -> ()  [unwired: 1 out]
                                n127 = call "GetActImgMem.vi"("Camera Handle In"=w257) -> ("Image Memory Out"=w258:u8[])  [unwired: 1 in, 9 out]
                                }
                                frame #1 {
                                n128 = Unbundle(w261) -> ("Height"=w260:i32, "Width"=w259:i32)
                                n129 = Reshape Array(w263, w260, w259) -> (w262:u8[][])
                                }
                                }
                                n130 = local read "templateSiz"() -> (w249:dbl)
                                n131 = local read "add Factor"() -> (w250:dbl)
                                n132 = local read "Index #"() -> (w245:i32)
                                n133 = local read "centerx"() -> (w252:dbl)
                                n134 = local read "centery"() -> (w251:dbl)
                                n135 = script code="windowsiz = templateSiz;\nxrange = centerx-windowsiz:centerx+windowsiz;\nyrange = centery-windowsiz:centery+windowsiz;\ntemplateImg = img(yrange,xrange);\n    \naxialPath = fullfile(dirpath,['AxialImageCalibration_' num2str(index)]);     \nmkdir(axialPath);    \ndlmwrite(fullfile(axialPath,'templateImg.txt'),templateImg,'delimiter','\\t','newline','pc');\n    \nfigure(1); clf;     \nimagesc(templateImg); colormap gray;\ntitle(num2str(i));   \nprint('-djpeg',fullfile(axialPath,'templateImg'));\n  \nclose all;"("img"=w254, "centerx"=w252, "centery"=w251, "dirpath"=w253, "addFactor"=w250, "templateSiz"=w249, "index"=w245) -> ("templateImg"=→"ztemplateImg":dbl[][])  [unwired: 1 in, 1 out]
                              }
                              frame #2 {
                                w268 = u16 2 items=["X", "Y", "Z"] ("Axis")
                                n136 = Wait (ms)(milliseconds to wait=u32 500) -> ()  [unwired: 1 out]
                                n137 = call "sub vi - Move Piezo Stage (Single).vi"("frequency"=0.5, "Desired Position (um)"=w266, "Axis"=w268) -> ("Z Position"=w265:dbl)  [unwired: 2 out]
                                n138 = local write "Z Position"(w265) -> ()
                              }
                            }
                          }
                          frame #1 {
                            # "Get the axial Correlation calibration"
                            n139 = call "sub vi - ReadPosition.vi"() -> ("Z Position"=w278:dbl)  [unwired: 6 in, 5 out]
                            n140 = script code="start = zpos-windowsiz;\nfinish = zpos+windowsiz;\n\nrange = start:stepsiz:finish;\nnumSteps = length(range)-1;"("zpos"=w278, "stepsiz"="z-stepsiz (um)", "windowsiz"="z-window (um)") -> ("numSteps"=w275:dbl, "range"=w269:dbl[])  [unwired: 1 in, 1 out]
                            "Total Steps" <- w275
                            n141 = while {
                              tunnel: w275 -> [w290]
                              tunnel: w269 -> [w288] mode=indexing
                              tunnel: w269 -> [w286]
                              tunnel: w274 -> [w285]
                              tunnel: w273 -> [w284]
                              tunnel: w272 -> [w283]
                              shift-right: [w282] -> w270
                              shift-left: dbl[] [] -> [w280]
                              i -> [w289]
                              stop <- w287 stop-if-true
                              n142 = Greater Or Equal?(x=w289, y=w290) -> (x >= y?=w287:bool)
                              n143 = stacked-sequence {
                                tunnel: w289 -> [_ w308]
                                tunnel: w288 -> [w292 _]
                                tunnel: w286 -> [_ _]
                                tunnel: w285 -> [_ w301]
                                tunnel: w284 -> [_ w300]
                                tunnel: w283 -> [_ w299]
                                tunnel: [_ w298] -> w281
                                frame #0 {
                                w294 = u16 2 items=["X", "Y", "Z"] ("Axis")
                                n144 = Wait (ms)(milliseconds to wait=u32 100) -> ()  [unwired: 1 out]
                                n145 = call "sub vi - Move Piezo Stage (Single).vi"("frequency"=0.5, "Desired Position (um)"=w292, "Axis"=w294) -> ("Z Position"=w291:dbl)  [unwired: 2 out]
                                n146 = local write "Z Position"(w291) -> ()
                                }
                                frame #1 {
                                n147 = flat-sequence {
                                tunnel: [w313] -> w311
                                tunnel: w299 -> [w312]
                                tunnel: w311 -> [w318]
                                tunnel: [w317] -> w310
                                tunnel: w300 -> [w316]
                                frame #0 {
                                n148 = call "GetActImgMem.vi"("Camera Handle In"=w312) -> ("Image Memory Out"=w313:u8[])  [unwired: 1 in, 9 out]
                                }
                                frame #1 {
                                n149 = Unbundle(w316) -> ("Height"=w315:i32, "Width"=w314:i32)
                                n150 = Reshape Array(w318, w315, w314) -> (w317:u8[][])
                                }
                                }
                                n151 = Wait Until Next ms Multiple(millisecond multiple=u32 500) -> ()  [unwired: 1 out]
                                n152 = local read "ztemplateImg"() -> (w297:dbl[][])
                                n153 = local read "Index #"() -> (w296:i32)
                                n154 = local read "templateSiz"() -> (w302:dbl)
                                n155 = local read "add Factor"() -> (w303:dbl)
                                n156 = local read "centerx"() -> (w305:dbl)
                                n157 = local read "centery"() -> (w304:dbl)
                                n158 = Boolean To (0,1)(Boolean="Save Data") -> (0, 1=w306:i16)
                                n159 = script code="windowsiz = templateSiz + addFactor;\nxrange = centerx-windowsiz:centerx+windowsiz;\nyrange = centery-windowsiz:centery+windowsiz;\nimg2 = img(yrange,xrange);\n\nif saveData == 1\n    axialPath = fullfile(dirpath,['AxialImageCalibration_' num2str(index)]); \n    mkdir(axialPath);\n    dlmwrite(fullfile(axialPath,[num2str(i) '.txt']),img2,'delimiter','\\t','newline','pc');\n    figure(1); clf; \n    imagesc(img2); colormap gray;\n    title(num2str(i));\n    print('-djpeg',fullfile(axialPath,num2str(i)));\nend\n[xoffset yoffset max_C] = FindCorr(templateImg,img2,templateSiz,addFactor);\n            \nclose all;"("img"=w310, "centerx"=w305, "centery"=w304, "dirpath"=w301, "i"=w308, "saveData"=w306, "addFactor"=w303, "templateSiz"=w302, "templateImg"=w297, "index"=w296) -> ("max_C"=w298:dbl)  [unwired: 1 in, 1 out]
                                }
                              }
                              n160 = Build Array (concatenate)(w280, w281) -> (w282:dbl[])
                              "Step" <- w289
                            }
                            "?" <- TRUE
                          }
                          frame #2 {
                            # "find the sensitivity"
                            n161 = local read "Save Data"() -> (w323:bool)
                            n162 = local read "z-stepsiz (um)"() -> (w321:dbl)
                            n163 = local read "z-window (um)"() -> (w328:dbl)
                            n164 = local read "Index #"() -> (w319:i32)
                            n165 = Boolean To (0,1)(Boolean=w323) -> (0, 1=w324:i16)
                            n166 = script code="lockIndex =windowsiz/stepsiz+1;\n%zsetpoint = z(lockIndex);\nsetpoint = C(lockIndex);\nrange =lockIndex-2:lockIndex+2;\nx = z(range);        \ny = C(range);        \nf = fittype('a*x+b');       \n [c gof] = fit(x',y',f,'startpoint',[-1 1]);\nslope = c.a;\n       \nfigure(1); clf; hold on; box on;        \nplot(z,C,'linewidth',2);\nx = z(range);\ny = c(x')';\nplot(x,y,'r','linewidth',2);        \nxlabel('Z position (nm)','fontsize',14);\nylabel('Normalized Cross-Correlation','fontsize',14);\ntitle(['Axial Displacement Signal (' num2str(c.a)  ')'],'fontsize',16,'fontweight','b');\n\naxialPath = fullfile(dirpath,['AxialImageCalibration_' num2str(index)]); \nprint('-djpeg',fullfile(axialPath,'z-CalibrationFit'));\ndlmwrite(fullfile(axialPath, 'axialPositions.txt'),axialpos,'delimiter','\\t','newline','pc');"("z"=w320, "C"=w322, "windowsiz"=w328, "dirpath"=w327, "saveData"=w324, "axialpos"=w320, "stepsiz"=w321, "index"=w319) -> ("setpoint"=→"z-setpoint":dbl, "slope"=→"z-sensitivity":dbl)  [unwired: 1 in, 1 out]
                          }
                          frame #3 {
                            w333 = u16 2 items=["X", "Y", "Z"] ("Axis")
                            n167 = call "sub vi - Move Piezo Stage (Single).vi"("frequency"=0.5, "Desired Position (um)"=w331, "Axis"=w333) -> ("Z Position"=w330:dbl)  [unwired: 2 out]
                            n168 = local write "Z Position"(w330) -> ()
                            n169 = Wait Until Next ms Multiple(millisecond multiple=u32 500) -> ()  [unwired: 1 out]
                          }
                        }
                      }
                    }
                    "Image" <- w207
                  }
                }
              }
              frame #4 {
                # "monitor the drift and correct with a PID feedback"
                n170 = local read "Monitor Drift"() -> (w334:bool)
                n171 = local read "status"() -> (w342:dbl)
                n172 = Equal?(x=w342, y=1.0) -> (x = y?=w343:bool)
                n173 = And(x=w343, y=w334) -> (x .and. y?=w344:bool)
                n174 = case shown="True" w344 {
                  tunnel: w340 -> [_ w371]
                  tunnel: w339 -> [_ w370]
                  tunnel: w335 -> [_ w348]
                  frame False {
                  }
                  frame True {
                    w355 = dbl[] []
                    w360 = 0.0
                    w358 = 0.0
                    n175 = call "sub vi - ReadPosition.vi"() -> ("Z Position"=w356:dbl, "Y Voltage"=w357:dbl)  [unwired: 10 out]
                    n176 = while {
                      tunnel: w371 -> [w420]
                      tunnel: w370 -> [w414]
                      shift-right: [w409] -> w367
                      shift-left: dbl[] [] -> [w419]
                      shift-right: [w410] -> w366
                      shift-left: dbl[] [] -> [w418]
                      shift-right: [w374] -> _
                      shift-left: w358 -> [w416]
                      shift-right: [w408] -> _
                      shift-left: w360 -> [w415]
                      shift-right: [w403] -> w361
                      shift-left: dbl[] [] -> [w377]
                      shift-right: [w407] -> _
                      shift-left: w360 -> [w406]
                      shift-right: [w404] -> w359
                      shift-left: w355 -> [w405]
                      shift-right: [w398] -> _
                      shift-left: w358 -> [w400]
                      shift-right: [w397] -> _
                      shift-left: w358 -> [w399]
                      shift-right: [w375] -> _
                      shift-left: w357 -> [w396]
                      shift-right: [w376] -> _
                      shift-left: w356 -> [w395]
                      shift-right: [w382] -> _
                      shift-left: w355 -> [w389]
                      shift-right: [w381] -> _
                      shift-left: w355 -> [w388]
                      shift-right: [w380] -> _
                      shift-left: w355 -> [w387]
                      shift-right: [w379] -> _
                      shift-left: w355 -> [w386]
                      tunnel: [w376] -> w345 mode=indexing
                      tunnel: [w375] -> w346 mode=indexing
                      tunnel: [w374] -> w347 mode=indexing
                      i -> [w401]
                      stop <- "?" stop-if-true
                      n177 = for {
                        N: "# Average" -> [_]
                        tunnel: w420 -> [w451]
                        tunnel: [w449] -> w391 mode=indexing
                        tunnel: w414 -> [w448]
                        tunnel: [w447] -> w390 mode=indexing
                        tunnel: [w442] -> w392 mode=indexing
                        tunnel: w401 -> [w441]
                        tunnel: w400 -> [w438]
                        tunnel: w399 -> [w437]
                        tunnel: [w436] -> w398
                        tunnel: [w435] -> w397
                        tunnel: [w434] -> w394
                        n178 = flat-sequence {
                          tunnel: [w463] -> w458
                          tunnel: w448 -> [w462]
                          tunnel: w458 -> [w468]
                          tunnel: w451 -> [w467]
                          tunnel: [w464] -> w443
                          frame #0 {
                            n179 = local read "Exposure time 2"() -> (w460:dbl)
                            n180 = call "GetActImgMem.vi"("Camera Handle In"=w462) -> ("Image Memory Out"=w463:u8[])  [unwired: 1 in, 9 out]
                            n181 = Add(x=w460, y=50.0) -> (x+y=w461:dbl)
                            n182 = Wait Until Next ms Multiple(millisecond multiple=w461) -> ()  [unwired: 1 out]
                          }
                          frame #1 {
                            n183 = Unbundle(w467) -> ("Height"=w466:i32, "Width"=w465:i32)
                            n184 = Reshape Array(w468, w466, w465) -> (w464:u8[][])
                          }
                        }
                        n185 = local read "z-setpoint"() -> (w446:dbl)
                        n186 = local read "scale"() -> (w455:dbl)
                        n187 = local read "add Factor"() -> (w456:dbl)
                        n188 = local read "templateSiz"() -> (w457:dbl)
                        n189 = local read "lockinImg"() -> (w454:dbl[][])
                        n190 = local read "centerx"() -> (w453:dbl)
                        n191 = local read "centery"() -> (w452:dbl)
                        n192 = local write "Image"(w443) -> ()
                        n193 = local read "ztemplateImg"() -> (w444:dbl[][])
                        n194 = local read "z-sensitivity"() -> (w445:dbl)
                        n195 = Boolean To (0,1)(Boolean="reset") -> (0, 1=w439:i16)
                        n196 = script code="xfeedback = 0;\n    yfeedback = 0;\n    zfeedback = 0;\n    status = 0;\ntry\nwindowsiz = templateSiz + addFactor;\nxrange = round(centerx-windowsiz:centerx+windowsiz);\nyrange = round(centery-windowsiz:centery+windowsiz);\nnewImg = img(yrange,xrange);\n\n[xoffset yoffset max_c] = FindPixelOffset(templateImg,newImg,templateSiz,addFactor,scale);\n[xpeak ypeak max_c] = FindCorr(ztemplateImg,newImg,templateSiz,addFactor);\nslope = -slope;\nif i == 0\n     zsetpoint = max_c;\nend\n if reset == 1\n     xinitial = xoffset;\n     yinitial = yoffset;\n     zsetpoint = max_c;\nend\nxfeedback = (xoffset - xinitial)/pixels2um*1000;    \nyfeedback = (yoffset - yinitial)/pixels2um*1000;\nzfeedback = (max_c - zsetpoint)/slope*1000;\n\n%if xfeedback > 100\n%xfeedback = 100;\n%elseif xfeedback < -100\n%xfeedback = -100;\n%end\n%if yfeedback > 20\n%yfeedback = 20;\n%elseif yfeedback < -20\n%yfeedback = -20;\n%end\n%if zfeedback >30\n%zfeedback =30;\n%elseif zfeedback < -30\n%zfeedback = -30;\n%end\n\nstatus = 1;\ncatch\n    xfeedback = 0;\n    yfeedback = 0;\n    zfeedback = 0;\n    status = 0;\nend"("img"=w443, "templateSiz"=w457, "addFactor"=w456, "scale"=w455, "templateImg"=w454, "centerx"=w453, "centery"=w452, "xinitial"=w438, "yinitial"=w437, "pixels2um"="pixels2um", "zsetpoint2"=w446, "slope"=w445, "ztemplateImg"=w444, "i"=w441, "reset"=w439) -> ("xfeedback"=w447:dbl, "yfeedback"=w449:dbl, "zfeedback"=w442:dbl, "xinitial"=w436:dbl, "yinitial"=w435:dbl, "status"=w434:dbl)  [unwired: 1 in, 1 out]
                        "# of frames" <- w441
                      }
                      n197 = call <vilib>:"Mean.vi"("X"=w392) -> ("mean"=w385:dbl)  [unwired: 1 out]
                      n198 = call <vilib>:"Mean.vi"("X"=w390) -> ("mean"=w384:dbl)  [unwired: 1 out]
                      n199 = call <vilib>:"Mean.vi"("X"=w391) -> ("mean"=w383:dbl)  [unwired: 1 out]
                      n200 = Build Array (concatenate)(w405, w385) -> (w404:dbl[])
                      n201 = Build Array (concatenate)(w418, w383) -> (w410:dbl[])
                      n202 = Build Array (concatenate)(w419, w384) -> (w409:dbl[])
                      n203 = case shown="1" w394 {
                        tunnel: w383 -> [w470 w487]
                        tunnel: w416 -> [w473 w486]
                        tunnel: w415 -> [_ w485]
                        tunnel: [w472 w484] -> w374
                        tunnel: [w473 w483] -> w408
                        tunnel: w384 -> [_ w482]
                        tunnel: [w474 w481] -> w407
                        tunnel: w406 -> [w474 w480]
                        tunnel: w385 -> [w471 w479]
                        tunnel: [w470 w478] -> w375
                        tunnel: w396 -> [_ w477]
                        tunnel: [w471 w476] -> w376
                        tunnel: w395 -> [w472 w475]
                        frame 0, Default {
                          "Boolean" <- TRUE ("Boolean")
                        }
                        frame 1 {
                          n204 = stacked-sequence {
                            tunnel: w482 -> [w491 _ _]
                            tunnel: w487 -> [_ w512 _]
                            tunnel: [w490 _ _] -> w484
                            tunnel: w486 -> [w489 _ _]
                            tunnel: [_ w511 _] -> w483
                            tunnel: w485 -> [_ w510 _]
                            tunnel: w479 -> [_ _ w533]
                            tunnel: [_ _ w532] -> w481
                            tunnel: w480 -> [_ _ w531]
                            tunnel: [_ w508 _] -> w478
                            tunnel: w477 -> [_ w507 _]
                            tunnel: [_ _ w530] -> w476
                            tunnel: w475 -> [_ _ w529]
                            frame #0 {
                              n205 = case shown="False" "fix x" {
                                tunnel: w491 -> [_ w498]
                                tunnel: [0.0 w506] -> w490
                                tunnel: w489 -> [_ w499]
                                frame False {
                                }
                                frame True {
                                w496 = u16 0 items=["X", "Y", "Z"] ("Axis")
                                n206 = call "sub vi - ReadPosition.vi"() -> ("X Position"=w494:dbl)  [unwired: 11 out]
                                n207 = Divide(x=w498, y=1000.0) -> (x/y=w500:dbl)
                                n208 = Add(x=w499, y=w500) -> (x+y=w506:dbl)
                                n209 = Multiply(x="P (xy)", y=w500) -> (x*y=w502:dbl)
                                n210 = Multiply(x=w506, y="I (xy)") -> (x*y=w501:dbl)
                                n211 = Add(x=w502, y=w501) -> (x+y=w497:dbl)
                                n212 = Add(x=w494, y=w497) -> (x+y=w495:dbl)
                                n213 = call "sub vi - Move Piezo Stage (Single).vi"("Desired Position (um)"=w495, "Axis"=w496) -> ("X Position"=w493:dbl)  [unwired: 1 in, 2 out]
                                n214 = local write "X Position"(w493) -> ()
                                }
                              }
                            }
                            frame #1 {
                              n215 = case shown="True" "fix y" {
                                tunnel: w512 -> [_ w528]
                                tunnel: [0.0 w527] -> w511
                                tunnel: w510 -> [_ w526]
                                tunnel: [w513 w516] -> w508
                                tunnel: w507 -> [w513 _]
                                frame False {
                                }
                                frame True {
                                w517 = u16 1 items=["X", "Y", "Z"] ("Axis")
                                (unwired) u16 1 items=["X", "Y", "Z"] ("Axis")
                                n216 = local read "P (xy)"() -> (w523:dbl)
                                n217 = local read "I (xy)"() -> (w521:dbl)
                                n218 = Divide(x=w528, y=1000.0) -> (x/y=w520:dbl)
                                n219 = call "sub vi - ReadPosition.vi"() -> ("Y Position"=w518:dbl)  [unwired: 11 out]
                                n220 = Add(x=w520, y=w526) -> (x+y=w527:dbl)
                                n221 = Multiply(x=w527, y=w521) -> (x*y=w519:dbl)
                                n222 = Multiply(x=w520, y=w523) -> (x*y=w522:dbl)
                                n223 = Add(x=w522, y=w519) -> (x+y=w525:dbl)
                                n224 = Add(x=w518, y=w525) -> (x+y=w516:dbl)
                                n225 = call "sub vi - Move Piezo Stage (Single).vi"("Desired Position (um)"=w516, "Axis"=w517) -> ("Y Position"=w515:dbl)  [unwired: 1 in, 2 out]
                                n226 = local write "Y Position"(w515) -> ()
                                }
                              }
                            }
                            frame #2 {
                              n227 = case shown="True" "fix z" {
                                tunnel: w533 -> [_ w545]
                                tunnel: [w536 w544] -> w532
                                tunnel: w531 -> [w536 w543]
                                tunnel: [w535 w539] -> w530
                                tunnel: w529 -> [w535 _]
                                frame False {
                                }
                                frame True {
                                w542 = u16 2 items=["X", "Y", "Z"] ("Axis")
                                n228 = Divide(x=w545, y=1000.0) -> (x/y=w541:dbl)
                                n229 = call "sub vi - ReadPosition.vi"() -> ("Z Position"=w537:dbl)  [unwired: 11 out]
                                n230 = Add(x=w541, y=w543) -> (x+y=w544:dbl)
                                n231 = Multiply(x="P (z)", y=w541) -> (x*y=w548:dbl)
                                n232 = Multiply(x=w544, y="I (z)") -> (x*y=w547:dbl)
                                n233 = Add(x=w548, y=w547) -> (x+y=w546:dbl)
                                n234 = Add(x=w537, y=w546) -> (x+y=w539:dbl)
                                n235 = call "sub vi - Move Piezo Stage (Single).vi"("Desired Position (um)"=w539, "Axis"=w542) -> ("Z Position"=w538:dbl)  [unwired: 1 in, 2 out]
                                n236 = local write "Z Position"(w538) -> ()
                                }
                              }
                            }
                          }
                        }
                      }
                      n237 = call "Elapsed Time2"("Time Target (s)"=10000.0) -> ("Elapsed Time (s)"=w372:dbl)  [unwired: 11 in, 7 out]
                      n238 = case shown="False" "Reset" {
                        tunnel: w389 -> [w432 _]
                        tunnel: w388 -> [w431 _]
                        tunnel: w387 -> [w430 _]
                        tunnel: w386 -> [w429 _]
                        tunnel: w385 -> [w428 _]
                        tunnel: w372 -> [w427 _]
                        tunnel: w384 -> [w426 _]
                        tunnel: w383 -> [w425 _]
                        tunnel: [w424 w433] -> w382
                        tunnel: [w423 w433] -> w381
                        tunnel: [w422 w433] -> w380
                        tunnel: [w421 w433] -> w379
                        frame False {
                          n239 = Build Array (concatenate)(w431, w427) -> (w423:dbl[])
                          n240 = Build Array (concatenate)(w432, w428) -> (w424:dbl[])
                          n241 = Build Array (concatenate)(w430, w426) -> (w422:dbl[])
                          n242 = Build Array (concatenate)(w429, w425) -> (w421:dbl[])
                        }
                        frame True {
                          w433 = dbl[] []
                        }
                      }
                      n243 = Bundle(w381, w380) -> (w412:cluster{dbl[], dbl[]})  [unwired: 1 in]
                      n244 = Bundle(w381, w382) -> (w402:cluster{dbl[], dbl[]})  [unwired: 1 in]
                      n245 = Bundle(w381, w379) -> (w411:cluster{dbl[], dbl[]})  [unwired: 1 in]
                      n246 = Build Array(w412, w411, w402) -> (→"?":cluster{dbl[], dbl[]}[])
                      n247 = Build Array (concatenate)(w377, w372) -> (w403:dbl[])
                    }
                    n248 = Build Array(w361, w367, w366, w359, w347, w346, w345) -> (w365:dbl[][])
                    n249 = Number To Decimal String(number="Index #") -> (decimal integer string=w350:string)  [unwired: 1 out]
                    n250 = call "Convert to Dynamic Data"("2D Array"=w365) -> ("Dynamic Data Type"=w364:dynamicdata)  [unwired: 3 in]
                    n251 = Concatenate Strings(w348, "Filename", "_" ("string"), w350, ".txt" ("string")) -> (w349:string)
                    n252 = String To Path(string=w349) -> (path=w363:path)
                    n253 = call "Write To Measurement File"("Signals"=w364, "Filename"=w363) -> ()  [unwired: 15 in, 3 out]
                  }
                }
                n254 = local write "fix y"(FALSE ("fix y")) -> ()
                n255 = local write "fix z"(FALSE ("fix z")) -> ()
                n256 = local write "fix x"(FALSE ("fix x")) -> ()
              }
              frame #5 {
                n257 = local write "Select Lockin \n(autofocus)"(FALSE ("Select Lockin \n(autofocus)")) -> ()
                n258 = local write "Select Lockin\n(Drift Bead)"(FALSE ("Select Lockin\n(Drift Bead)")) -> ()
                n259 = local write "Center Piezo"(FALSE ("Center Piezo")) -> ()
                n260 = local write "Monitor Drift"(FALSE ("Monitor Drift")) -> ()
                n261 = local write "autofocus"(FALSE ("autofocus")) -> ()
              }
            }
          }
        }
      }
    }
    frame #1 {
      # "Stop Capture"
      n262 = call "StopLiveVideo.vi"("Camera Handle In"=w558) -> ("error out"=w559:errorcluster, "Camera Handle Out"=w560:u32)  [unwired: 2 in, 7 out]
      n263 = local write item#9(FALSE ("Template")) -> ()
      n264 = local write item#43(FALSE) -> ()
      n265 = call "ExitCamera.vi"("error in"=w559, "Camera Handle In"=w560) -> ()  [unwired: 10 out]
    }
  }
